vi "FRCts20_Backend_Update_S3_API.vi"(6 "Message Attributes":T1, 8 "error in (no error)":errorcluster, 10 "Data":string, 11 "Engine_Refnums":T2) -> (0 "error out":errorcluster)   [LabVIEW 2014, in "FRCts20_Backend_Engine.lvlib"]
uses:
  FRCts20_Backend_Engine.lvlib
  FRCts20_Backend_EngineRefnums.ctl
  INI_Accessor/FRCts20_Backend_INI Controller.lvclass
  Dependencies/AMC/_SubVIs/TypeDefs/Message Queue.ctl
  Dependencies/AMC/_SubVIs/TypeDefs/Message.ctl
  Dependencies/Keyed Array/KeyedArray.ctl
  <vilib>/addons/database/Connection.llb/Conn ObjectReference.ctl
  FRCts20_Backend_FGVOperation.ctl
  FRCts20_Backend_API/FRCts20_Backend_API_S3.ctl
  FRCts20_Backend_API/FRCts20_Backend_API_Command_Team.ctl
  FRCts20_Backend_API/FRCts20_Backend_API_Team.ctl
  FRCts20_Backend_API/FRCts20_Backend_API_SW.ctl
  FRCts20_Backend_API/FRCts20_Backend_API_Status.ctl
  AWS Credentials.vi
  FRCts20_Backend_API/FRCts20_Backend_API_Team.vi
  FRCts20_Backend_API/FRCts20_Backend_API.lvlib
  <vilib>/National Instruments/NI Amazon Web Services (AWS) Toolkit for LabVIEW/S3/vi source/LV Interface for Amazon S3.lvlib
  Dependencies/Keyed Array/Tools_KeyedArray.lvlib
  Dependencies/AMC/AMC.lvlib
  <vilib>/addons/database/NI_Database_API.lvlib
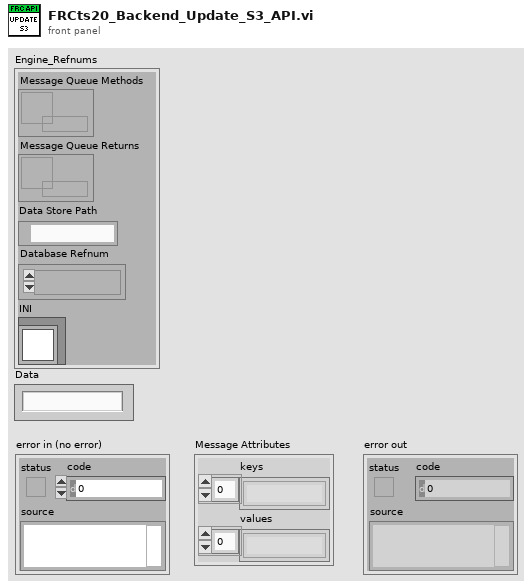
[diagram p1: front panel]
types:
  T1 = typedef "Tools_KeyedArray.lvlib/KeyedArray.ctl" = cluster{"keys":string[], "values":string[]}
  T2 = typedef "FRCts20_Backend_Engine.lvlib/FRCts20_Backend_EngineRefnums.ctl" = cluster{"Message Queue Methods":T3, "Message Queue Returns":T3, "Data Store Path":path, "Database Refnum":T4, "INI":refnum<class "FRCts20_Backend_INI Controller.lvclass">}
  T3 = typedef "AMC.lvlib/Message Queue.ctl" = refnum<queue>
  T4 = typedef "NI_Database_API.lvlib/Conn ObjectReference.ctl" = refnum<k1>
  T5 = typedef "FRCts20_Backend_API.lvlib/FRCts20_Backend_API_Team.ctl" = cluster{"Team Index":u32, "Team Number":u32, "Team Name":string, "Short Team Name":string, "Nick Name":string, "Robot Name":string, "City":string, "State":string, "Country":string, "Rookie Year":u32, "SWType":T6, "CAN":bool, "Vision":bool, "Kinect":bool, "Tags":string, "Avatar":string, "Request Array":cluster{"Request Index":u32, "Description":string, "Status":T7, "Open Date":timestamp, "Last Update":timestamp, "Close Date":timestamp}[], "Events Attending":cluster{"EventIndex":dbl, "EventName":string, "IsLive":bool}[], "APIReturn":string}
  T6 = typedef "FRCts20_Backend_API.lvlib/FRCts20_Backend_API_SW.ctl" = string
  T7 = typedef "FRCts20_Backend_API.lvlib/FRCts20_Backend_API_Status.ctl" = enum16{"Open", "In Work", "Closed"}
  T8 = typedef "FRCts20_Backend_API.lvlib/FRCts20_Backend_API_Command_Team.ctl" = string
  T9 = typedef "FRCts20_Backend_API.lvlib/FRCts20_Backend_API_S3.ctl" = cluster{"S3 API":string, "APIReturn":string, "Team Index":u32}
  T10 = typedef "FRCts20_Backend_Engine.lvlib/FRCts20_Backend_FGVOperation.ctl" = enum16{"Initialize", "EnqueueMessage", "EnqueueDataReturn", "FlushMessage", "FlushDataReturn"}
  T11 = typedef "LV Interface for Amazon S3.lvlib/AMZ_S3_AWS Credentials.ctl" = cluster{"Access Key":string, "Secret Key":string}
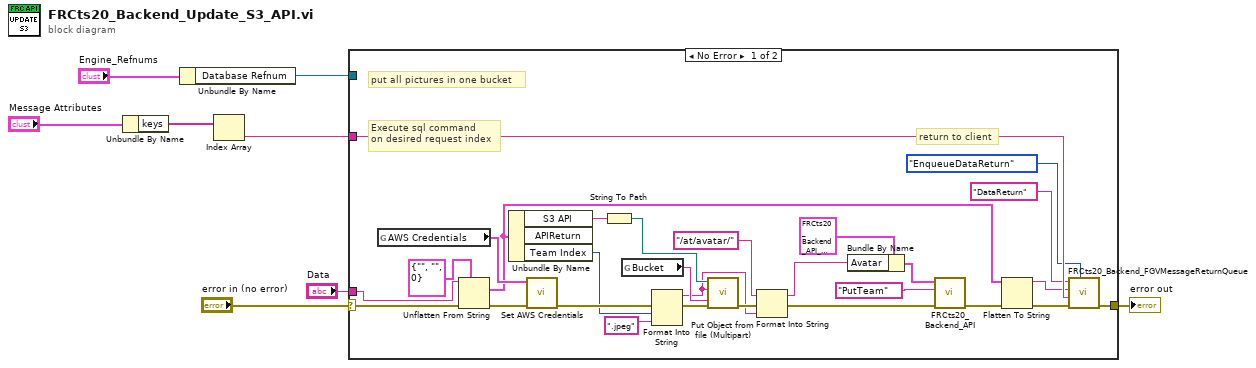
[diagram p0: block diagram]
diagram:
  n1 = Unbundle By Name("Message Attributes") -> ("keys"=w4:string[])
  n2 = Unbundle By Name("Engine_Refnums") -> ("Database Refnum"=w1:T4)
  n3 = Index Array(array=w4) -> (element=w3:string)  [unwired: 1 in]
  n4 = case shown="No Error" "error in (no error)" {
    selector: "error in (no error)" -> [w33 w37]
    tunnel: [w36 w37] -> w7
    tunnel: w1 -> [_ _]
    tunnel: "Data" -> [w34 _]
    tunnel: w3 -> [w35 _]
    frame No Error {
      # "put all pictures in one bucket"
      # "return to client"
      # "Execute sql command\non desired request index"
      n5 = global read "AWS Credentials.vi" "AWS Credentials"() -> (w26:T11)
      n6 = Unflatten From String(type=T9 {"S3 API"="", "APIReturn"="", "Team Index"=0} ("S3"), binary string=w34, error in (no error)=w33) -> (value=w14:T9, error out=w17:errorcluster)  [unwired: 2 in, 1 out]
      n7 = Unbundle By Name(w14) -> ("S3 API"=w23:string, "Team Index"=w20:u32)  [unwired: 1 out]
      n8 = call <vilib>:"Set AWS Credentials.vi"("error in (no error)"=w17, "AWS Credentials in"=w26) -> ("error out"=w22:errorcluster)  [unwired: 9 in]
      n9 = String To Path(string=w23) -> (path=w24:path)
      n10 = global read "AWS Credentials.vi" "Bucket"() -> (w25:string)
      n11 = Format Into String(error in=w22, w20, ".jpeg") -> (resulting string=w9:string, error out=w21:errorcluster)  [unwired: 2 in]
      n12 = call <vilib>:"Put Object from file (Multipart).vi"("error in (no error)"=w21, "Bucket"=w25, "Object path"=w9, "Local file path"=w24) -> ("error out"=w13:errorcluster)  [unwired: 5 in, 2 out]
      n13 = Format Into String(initial string="/at/avatar/" ("redirect URL"), error in=w13, w9) -> (resulting string=w11:string, error out=w12:errorcluster)  [unwired: 1 in]
      n14 = Bundle By Name(cluster=T5 {"Team Index"=0, "Team Number"=0, "Team Name"="", "Short Team Name"="", "Nick Name"="", "Robot Name"="", "City"="", "State"="", "Country"="", "Rookie Year"=0, "SWType"="", "CAN"=FALSE, "Vision"=FALSE, "Kinect"=FALSE, "Tags"="", "Avatar"="", "Request Array"=[], "Events Attending"=[], "APIReturn"=""} ("Team In"), "Avatar"=w11) -> (w15:T5)
      n15 = call-poly "FRCts20_Backend_API.vi"("error in (no error)"=w12, "Command"=T8 "PutTeam", "Team In"=w15) -> ("error out"=w18:errorcluster)  [unwired: 6 in, 2 out]
      n16 = Flatten To String(anything=w14, error in (no error)=w18) -> (data string=w28:string, error out=w27:errorcluster)  [unwired: 2 in, 1 out]
      n17 = call "FRCts20_Backend_FGVMessageReturnQueue.vi"("Operation"=FRCts20_Backend_FGVOperation."EnqueueDataReturn", "error in (no error)"=w27, "Key"=w35, "Message Value"=w28, "Message Name"="DataReturn") -> ("error out"=w36:errorcluster)  [unwired: 5 in, 1 out]
    }
    frame Error {
    }
  }
  "error out" <- w7
